vi "Name Globbing.vi"(10 "Index":i32, 11 "Tokens":string[](array[string])) -> (2 "Selected Tokens":string[](array[string]), 3 "WildCard?":bool)   [LabVIEW 2013]
panel:
  # "Globbing recognize 3 special characters\n/ - is the delimiter between name tokens\n* - is a wildcard for all choices\n| - delimites a set of choices"
  # "Examples:\n/LBCB2/Act/* asks for all actuator groups for LBCB2\n/LBCB1/Cart/Cmd|Disp asks for the cartesian commands and\ndisplacements for LBCB1."
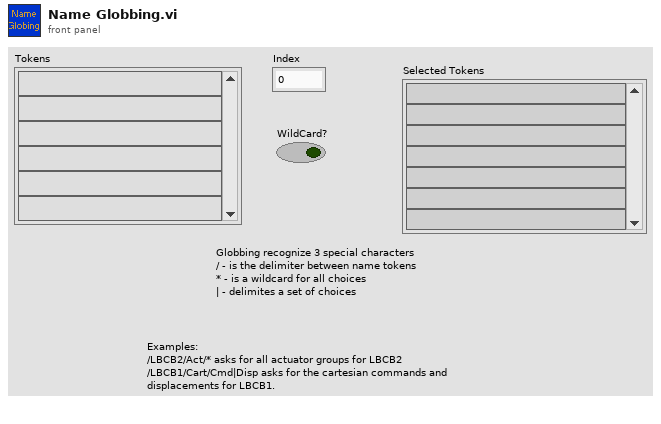
[diagram p1: front panel]
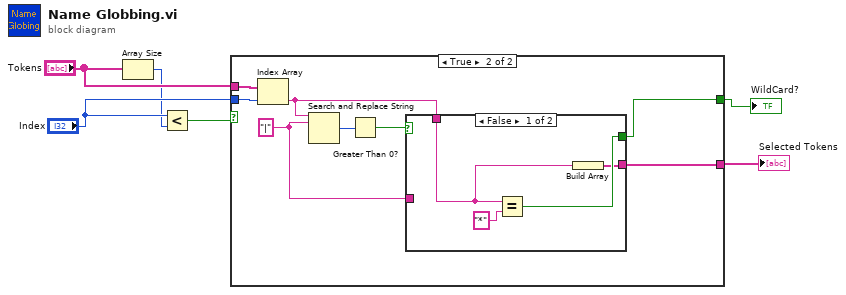
[diagram p0: block diagram]
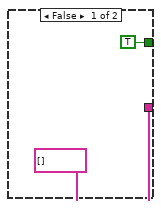
[diagram p2: hidden frame]
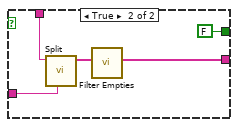
[diagram p3: hidden frame]
diagram:
  n1 = Array Size(array="Tokens") -> (size(s)=w3:i32)
  n2 = Less?(x="Index", y=w3) -> (x < y?=w2:bool)
  n3 = case shown="True" w2 {
    tunnel: [TRUE w9] -> w1
    tunnel: "Tokens" -> [_ w16]
    tunnel: "Index" -> [_ w15]
    tunnel: [string[] [] ("Out") w10] -> w6
    frame False {
    }
    frame True {
      w11 = "|" ("search string")
      n4 = Index Array(array=w16, index=w15) -> (element=w12:string)
      n5 = Search and Replace String(input string=w12, search string=w11) -> (number of replacements=w14:i32)  [unwired: 6 in, 3 out]
      n6 = Greater Than 0?(x=w14) -> (x > 0?=w13:bool)
      n7 = case shown="False" w13 {
        tunnel: w12 -> [w18 w25]
        tunnel: w11 -> [_ w24]
        tunnel: [w17 w22] -> w10
        tunnel: [w19 FALSE] -> w9
        frame False {
          n8 = Equal?(x=w18, y="*") -> (x = y?=w19:bool)
          n9 = Build Array(w18) -> (w17:string[])
        }
        frame True {
          n10 = call "Split.vi"("delimiter"=w24, "String"=w25) -> ("Array Result"=w23:string[])  [unwired: 9 in]
          n11 = call "Filter Empties.vi"("In"=w23) -> ("Out"=w22:string[])  [unwired: 10 in]
        }
      }
    }
  }
  "Selected Tokens" <- w6
  "WildCard?" <- w1
